vi "run.create.vi"(8 "error in":errorcluster, 9 "Start Time (now)":timestamp format="%<%x %.3X>T", 10 "Title":string, 11 "Nominal Client in":refnum<class "Nominal Client.lvclass">) -> (0 "error out":errorcluster, 2 "Run":refnum<class "Run.lvclass">, 3 "Nominal Client out":refnum<class "Nominal Client.lvclass">)   [LabVIEW 2020, in "Nominal Client.lvclass"]
doc: "Create a new run in Nominal.\nThrows if start is equal to or after end."
uses:
  Nominal Client.lvclass
  Run/Run.lvclass
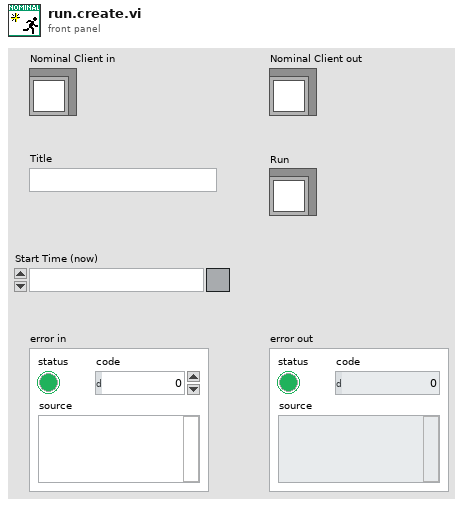
[diagram p1: front panel]
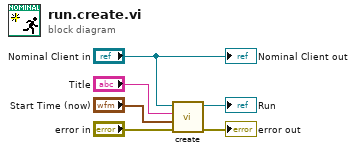
[diagram p0: block diagram]
diagram:
  n1 = call "create.vi"("error in (no error)"="error in", "Start Time"="Start Time (now)", "Title"="Title", "Nominal Client"="Nominal Client in") -> ("error out"=→"error out":errorcluster, "Run out"=→"Run":refnum<class "Run.lvclass">)  [unwired: 6 in]
  "Nominal Client out" <- "Nominal Client in"
